vi "TRITON_Read Field.vi"() -> (0 "Measurement":dbl, 2 "error out":errorcluster)   [LabVIEW 2021]
panel:
  out "output cluster":T1
  out "Response String":string
  in  "Mode":T2(ring)=enum."Immediate"
  in  "Bytes to Read":i32=5000
  in  "IP Address":string="192.168.0.2"
  in  "Remote Port":i32=33576
  in  "Timeout":i32=10000
  in  "error in (no error)":errorcluster
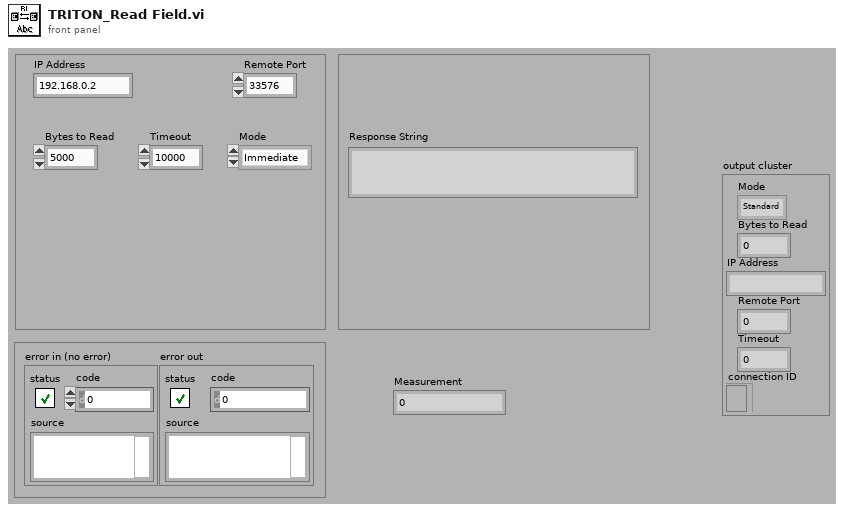
[diagram p1: front panel]
types:
  T1 = cluster{"Mode":enum16{"Standard", "Buffered", "CRLF", "Immediate"}, "Bytes to Read":i32, "IP Address":string, "Remote Port":i32, "Timeout":i32, "connection ID":refnum<k5>}
  T2 = enum16{"Standard", "Buffered", "CRLF", "Immediate"}
  T3 = cluster{"Mode":enum16{"Standard", "Buffered", "CRLF", "Immediate"}, "Bytes to Read":i32, "IP Address":string, "Remote Port":i32, "Timeout":i32}
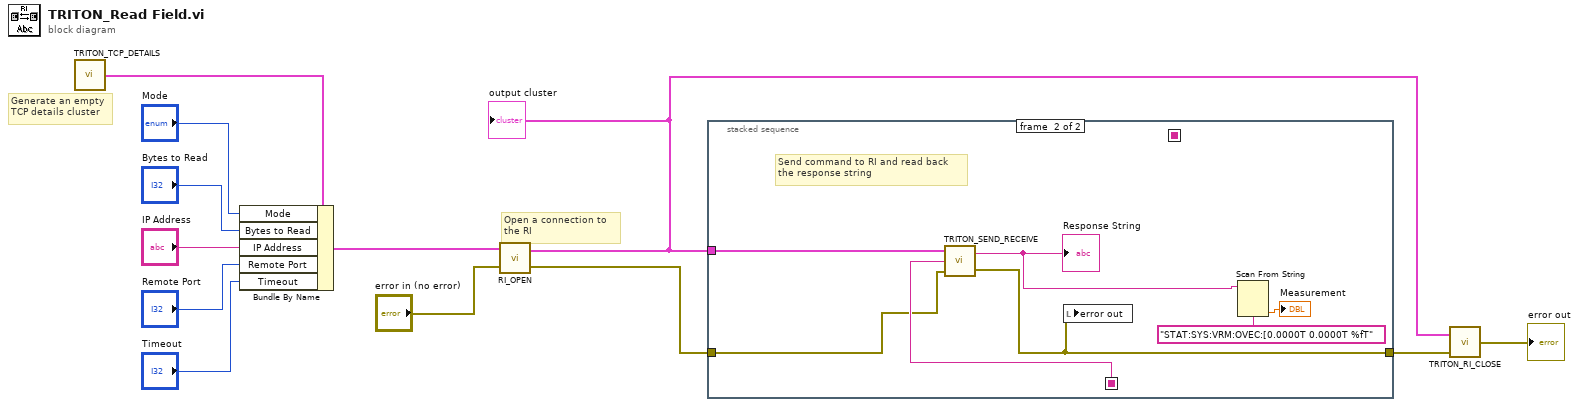
[diagram p0: block diagram]
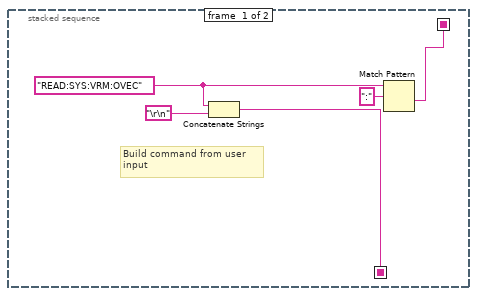
[diagram p2: hidden frame]
diagram:
  # "Open a connection to\nthe RI"
  # "Generate an empty\nTCP details cluster"
  n1 = call "TRITON_TCP_DETAILS.vi"() -> ("Cluster"=w12:T3)
  n2 = Bundle By Name(cluster=w12, "Mode"="Mode", "Bytes to Read"="Bytes to Read", "IP Address"="IP Address", "Remote Port"="Remote Port", "Timeout"="Timeout") -> (w10:T3)
  n3 = call "RI_OPEN.vi"("error in (no error)"="error in (no error)", "Cluster"=w10) -> ("error out"=w9:errorcluster, "output cluster"=w6:T1)
  "output cluster" <- w6
  n4 = stacked-sequence {
    seq-local: [w17 _] -> [_ w24]
    seq-local: [w14 _] -> [_ _]
    tunnel: w9 -> [_ w23]
    tunnel: [_ w22] -> w8
    tunnel: w6 -> [_ w21]
    frame #0 {
      w16 = "READ:SYS:VRM:OVEC" ("Command to send")
      # "Build command from user\ninput"
      n5 = Concatenate Strings(w16, "\r\n") -> (w17:string)
      n6 = Match Pattern(string=w16, regular expression=":") -> (after substring=w14:string)  [unwired: 1 in, 3 out]
    }
    frame #1 {
      # "Send command to RI and read back\nthe response string"
      n7 = call "TRITON_SEND_RECEIVE.vi"("error in (no error)"=w23, "Command String"=w24, "Communication Cluster"=w21) -> ("error out"=w22:errorcluster, "Response String"=w18:string)
      "Response String" <- w18
      n8 = local write "error out"(w22) -> ()
      n9 = Scan From String(format string="STAT:SYS:VRM:OVEC:[0.0000T 0.0000T %fT", input string=w18) -> (output 1=→"Measurement":dbl)  [unwired: 3 in, 3 out]
    }
  }
  n10 = call "TRITON_RI_CLOSE.vi"("error in (no error)"=w8, "Communication Cluster"=w6) -> ("error out"=→"error out":errorcluster)
